vi "Check stage contr is connected.vi"(8 "error in (no error)":errorcluster) -> (0 "error out":errorcluster)   [LabVIEW 2011]
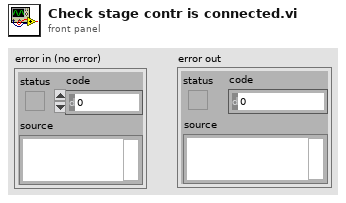
[diagram p1: front panel]
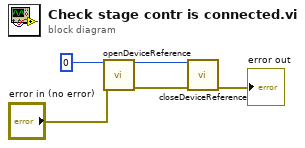
[diagram p0: block diagram]
diagram:
  n1 = call "openDeviceReference.vi"("deviceIndex"=0, "error in (no error)"="error in (no error)") -> ("reference"=w2:i32, "error out"=w3:errorcluster)  [unwired: 12 in]
  n2 = call "closeDeviceReference.vi"("reference"=w2, "error in (no error)"=w3) -> ("error out"=→"error out":errorcluster)  [unwired: 13 in]
